vi "InsertNewRoomEvent.vi"(8 "error in":errorcluster, 10 "EventTime":timestamp, 11 "Room.lvclass":refnum<class "Room.lvclass">) -> (0 "error out":errorcluster, 3 "Room out":refnum<class "Room.lvclass">)   [LabVIEW 2015, in "DatabaseApi.lvlib"]
uses:
  DatabaseApi.lvlib
  LVClasses/Room/Room.lvclass
  TypeDef/Room/RoomTableDbTableName.ctl
  TypeDef/Room/RoomTableColumnNames.ctl
  <vilib>/addons/database/Connection.llb/DB Tools Open Connec (Path).vi
  <vilib>/addons/database/NI_Database_API.lvlib
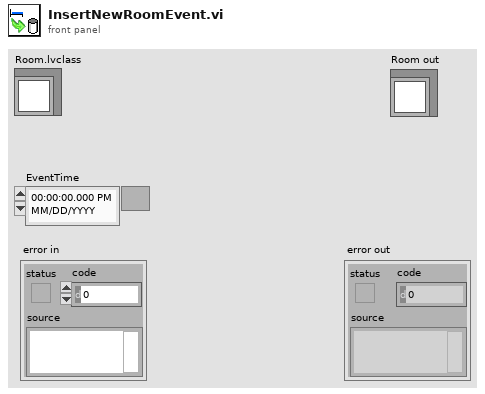
[diagram p1: front panel]
types:
  T1 = typedef "DatabaseApi.lvlib/RoomTableColumnNames.ctl" = string[]
  T2 = typedef "DatabaseApi.lvlib/RoomTableDbTableName.ctl" = string
  T3 = typedef "DatabaseApi.lvlib/RoomTableCluster.ctl" = cluster{"Room Number":i32, "EventTime":timestamp, "Flags":string, "BedVacant":i32, "InRoomPersonnel":string}
  T4 = typedef "NI_Database_API.lvlib/Conn ObjectReference.ctl" = refnum<k1>
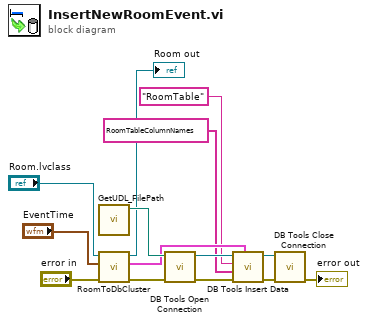
[diagram p0: block diagram]
diagram:
  n1 = call "GetUDL_FilePath.vi"() -> ("UDL file path"=w14:path)  [unwired: 11 in]
  n2 = call "RoomToDbCluster.vi"("error in"="error in", "EventTime"="EventTime", "Room.lvclass"="Room.lvclass") -> ("error out"=w7:errorcluster, "RoomEventCluster"=w3:T3, "Room out"=→"Room out":refnum<class "Room.lvclass">)  [unwired: 6 in]
  n3 = call-poly <vilib>:"DB Tools Open Connection.vi"("error in (no error)"=w7, "connection information"=w14) -> ("error out"=w10:errorcluster, "connection reference"=w11:T4)  [unwired: 6 in]
  n4 = call <vilib>:"DB Tools Insert Data.vi"("data"=w3, "error in (no error)"=w10, "columns"=T1 ["RoomNum", "EventTime", "Flags", "BedVacant", "InRoomPersonnel"] ("RoomTableColumnNames"), "table"=T2 "RoomTable" ("RoomTableName"), "connection reference"=w11) -> ("error out"=w12:errorcluster, "connection reference out"=w13:T4)  [unwired: 5 in]
  n5 = call <vilib>:"DB Tools Close Connection.vi"("error in (no error)"=w12, "connection reference"=w13) -> ("error out"=→"error out":errorcluster)  [unwired: 5 in]
